vi "Part 1.vi"(11 "Input":string) -> (3 "Output":i64)   [LabVIEW 2021]
uses:
  63b4fd2b-2e1b-4a3f-8c57-ff3ad7a63585.vi
  <userlib>/_OpenG.lib/string/string.llb/Convert EOLs (String)__ogtk.vi
panel:
  in  "Input 2":string
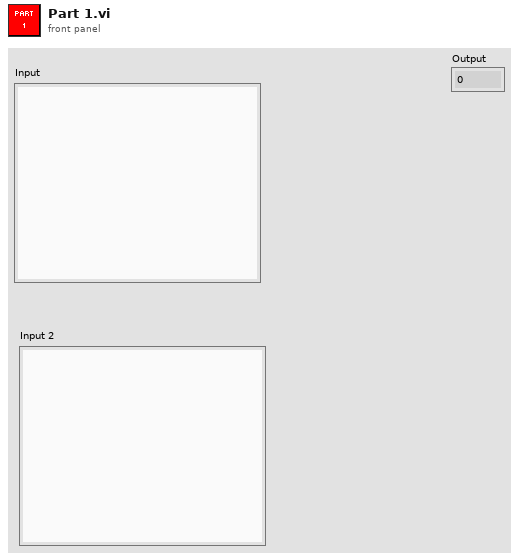
[diagram p1: front panel]
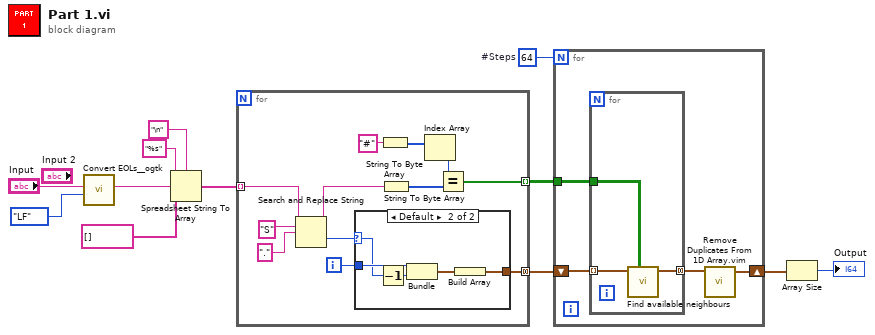
[diagram p0: block diagram]
diagram:
  w5 = 64  # #Steps
  n1 = call-poly <userlib>:"Convert EOLs__ogtk.vi"("Convert to:"=enum16{"CR", "LF", "CRLF"}."LF", "String in"="Input") -> ("String out"=w8:string)  [unwired: 9 in]
  n2 = Spreadsheet String To Array(delimiter (Tab)="\n", format string="%s", spreadsheet string=w8, array type (2D Dbl)=string[] []) -> (array=w6:string[])
  n3 = for {
    tunnel: w6 -> [w18] mode=indexing
    tunnel: [w20] -> w4 mode=indexing
    tunnel: [w13] -> w3 mode=concatenating
    i -> [w14]
    n4 = Search and Replace String(input string=w18, search string="S", replace string=".") -> (result string=w19:string, offset past replacement=w15:i32)  [unwired: 5 in, 2 out]
    n5 = case shown="Default" w15 {
      selector: w15 -> [_ w28]
      tunnel: w14 -> [_ w29]
      tunnel: [_ w25] -> w13
      frame -1 {
      }
      frame Default {
        n6 = Decrement(x=w28) -> (x-1=w27:i32)
        n7 = Bundle(w29, w27) -> (w26:cluster{i32, i32})  [unwired: 1 in]
        n8 = Build Array(w26) -> (w25:cluster{i32, i32}[])
      }
    }
    n9 = String To Byte Array(string="#") -> (unsigned byte array=w23:u8[])
    n10 = String To Byte Array(string=w19) -> (unsigned byte array=w21:u8[])
    n11 = Index Array(array=w23) -> (element=w22:u8)  [unwired: 1 in]
    n12 = Equal?(x=w22, y=w21) -> (x = y?=w20:bool[])
  }
  n13 = for {
    N: w5 -> [_]
    tunnel: w4 -> [w31]
    shift-right: [w33] -> w2
    shift-left: w3 -> [w32]
    n14 = for {
      tunnel: w32 -> [w34] mode=indexing
      tunnel: w31 -> [w36]
      tunnel: [w35] -> w30 mode=concatenating
      n15 = call "Find available neighbours.vi"("Grid"=w36, "Point"=w34) -> ("New points"=w35:cluster{i32, i32}[])  [unwired: 9 in]
    }
    n16 = call "Remove Duplicates From 1D Array.vim"("array"=w30) -> ("array with duplicates removed"=w33:cluster{i32, i32}[])  [unwired: 10 in]
  }
  n17 = Array Size(array=w2) -> (size(s)=→"Output":i32)
